vi "Day10-2.vi"() -> ()   [LabVIEW 2021]
uses:
  828a1bd3-9eb1-44bb-bb7d-0d736649e217.vi
  <vilib>/Comparison/Less/Less Functor/Less Functor.lvclass
panel:
  out "sum":i32
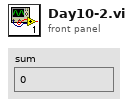
[diagram p1: front panel]
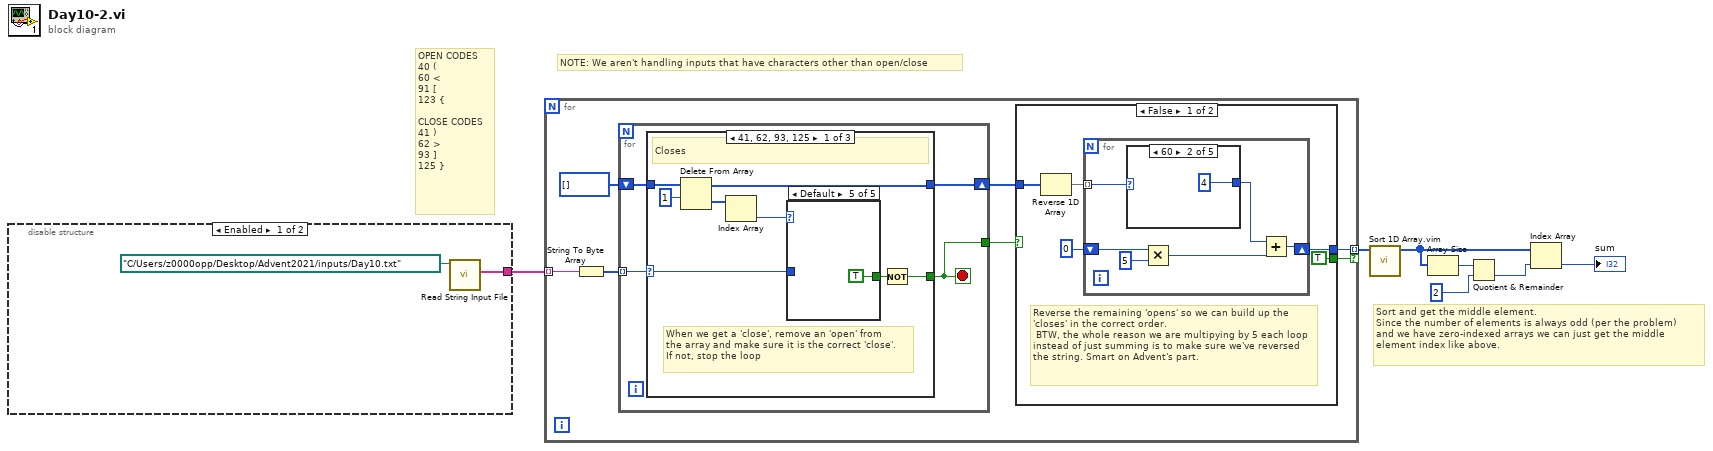
[diagram p0: block diagram]
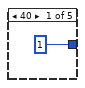
[diagram p2: hidden frame]
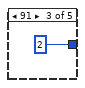
[diagram p3: hidden frame]
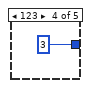
[diagram p4: hidden frame]
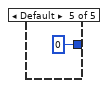
[diagram p5: hidden frame]
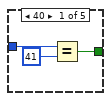
[diagram p7: hidden frame]
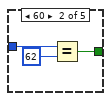
[diagram p8: hidden frame]
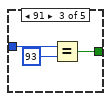
[diagram p9: hidden frame]
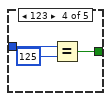
[diagram p10: hidden frame]
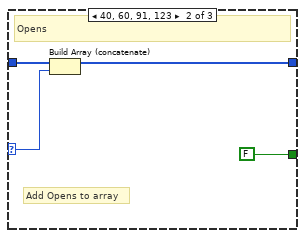
[diagram p11: hidden frame]
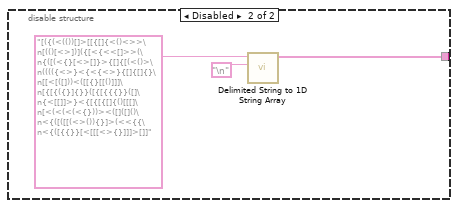
[diagram p13: hidden frame]
diagram:
  # "Sort and get the middle element.\nSince the number of elements is always odd (per the problem)\nand we have zero-indexed arrays we can just get the middle\nelement index like above."
  # "NOTE: We aren't handling inputs that have characters other than open/close"
  # "OPEN CODES\n40 (\n60 <\n91 [\n123 {\n\nCLOSE CODES\n41 )\n62 >\n93 ]\n125 }"
  n1 = disable-structure shown="Enabled" {
    disable-tunnel: [w8 w10] -> w7
    frame Enabled {
      n2 = call "Read String Input File.vi"("file path (dialog if empty)"=path "C:/Users/z0000opp/Desktop/Advent2021/inputs/Day10.txt") -> ("input values"=w8:string[])  [unwired: 10 in]
    }
    frame Disabled {
      n3 = call <vilib>:"Delimited String to 1D String Array.vi"("delimiter"="\n", "delimited string"="[({(<(())[]>[[{[]{<()<>>\n[(()[<>])]({[<{<<[]>>(\n{([(<{}[<>[]}>{[]{[(<()>\n(((({<>}<{<{<>}{[]{[]{}\n[[<[([]))<([[{}[[()]]]\n[{[{({}]{}}([{[{{{}}([]\n{<[[]]>}<{[{[{[]{()[[[]\n[<(<(<(<{}))><([]([]()\n<{([([[(<>()){}]>(<<{{\n<{([{{}}[<[[[<>{}]]]>[]]") -> ("string array"=w10:string[])  [unwired: 9 in]
    }
  }
  n4 = for {
    tunnel: w7 -> [w19] mode=indexing
    tunnel: [w15] -> w6 mode=indexing if=w13
    n5 = String To Byte Array(string=w19) -> (unsigned byte array=w18:u8[])
    n6 = for {
      tunnel: w18 -> [w37] mode=indexing
      shift-right: [w38] -> w16
      shift-left: u8[] [] -> [w39]
      tunnel: [w36] -> w14
      stop <- w36 stop-if-true
      n7 = case shown="41, 62, 93, 125" w37 {
        selector: w37 -> [w42 w63 _]
        tunnel: w39 -> [w47 w64 w65]
        tunnel: [w45 w62 w65] -> w38
        tunnel: [w40 FALSE _] -> w36
        frame 41, 62, 93, 125 {
          # "When we get a 'close', remove an 'open' from\nthe array and make sure it is the correct 'close'.\nIf not, stop the loop"
          # "Closes"
          n8 = Delete From Array(array=w47, length=1) -> (deleted portion=w44:u8[], array with subset deleted=w45:u8[])  [unwired: 1 in]
          n9 = Index Array(array=w44) -> (element=w43:u8)  [unwired: 1 in]
          n10 = case shown="Default" w43 {
            tunnel: w42 -> [w50 w53 w56 w59 _]
            tunnel: [w48 w51 w54 w57 TRUE] -> w41
            frame 40 {
              n11 = Equal?(x=w50, y=u8 41) -> (x = y?=w48:bool)
            }
            frame 60 {
              n12 = Equal?(x=w53, y=u8 62) -> (x = y?=w51:bool)
            }
            frame 91 {
              n13 = Equal?(x=w56, y=u8 93) -> (x = y?=w54:bool)
            }
            frame 123 {
              n14 = Equal?(x=w59, y=u8 125) -> (x = y?=w57:bool)
            }
            frame Default {
            }
          }
          n15 = Not(x=w41) -> (.not. x?=w40:bool)
        }
        frame 40, 60, 91, 123 {
          # "Add Opens to array"
          # "Opens"
          n16 = Build Array (concatenate)(w64, w63) -> (w62:u8[])
        }
        frame Default {
          # "ignore all other characters"
        }
      }
    }
    n17 = case shown="False" w14 {
      tunnel: w16 -> [w24 _]
      tunnel: [w21 _] -> w15
      tunnel: [TRUE _] -> w13
      frame False {
        # "Reverse the remaining 'opens' so we can build up the \n'closes' in the correct order.\n BTW, the whole reason we are multipying by 5 each loop instead of just summing is to make sure we've reversed the string. Smart on Advent's part."
        n18 = Reverse 1D Array(array=w24) -> (reversed array=w23:u8[])
        n19 = for {
          tunnel: w23 -> [w30] mode=indexing
          shift-right: [w25] -> w21
          shift-left: u64 0 -> [w29]
          n20 = case shown="60" w30 {
            tunnel: [u64 1 u64 4 u64 2 u64 3 u64 0] -> w26
            frame 40 {
            }
            frame 60 {
            }
            frame 91 {
            }
            frame 123 {
            }
            frame Default {
            }
          }
          n21 = Multiply(x=w29, y=u64 5) -> (x*y=w27:u64)
          n22 = Add(x=w26, y=w27) -> (x+y=w25:u64)
        }
      }
      frame True {
        # "we stopped early, so an invalid line"
      }
    }
  }
  n23 = call "Sort 1D Array.vim"("unsorted array"=w6) -> ("sorted array"=w4:u64[])  [unwired: 10 in]
  n24 = Array Size(array=w4) -> (size(s)=w5:i32)
  n25 = Quotient & Remainder(x=w5, y=2) -> (floor(x/y)=w1:i32)  [unwired: 1 out]
  n26 = Index Array(array=w4, index=w1) -> (element=→"sum":u64)
